vi "CheckCore.vi"(8 "error in (no error)":errorcluster, 9 "# of Refs":i32, 10 "References":refnum<vi>[](array[refnum]), 11 "Function in":refnum<class "Function.lvclass">) -> (0 "error out":errorcluster, 1 "Reject?":bool, 2 "dup References":refnum<vi>[](array[refnum]), 3 "Function out":refnum<class "Function.lvclass">)   [LabVIEW 2014, in "lvbuildsecurity.lvlib" / "Function.lvclass"]
uses:
  Function.lvclass
  Blacklist.lvclass/Blacklist.ctl
  ReadVIRefnum.vi
  ReadCLI.vi
  ReadItems.vi
  <vilib>/Wiresmith Technology/LabVIEW CLI/CLI Class/CLI.lvclass
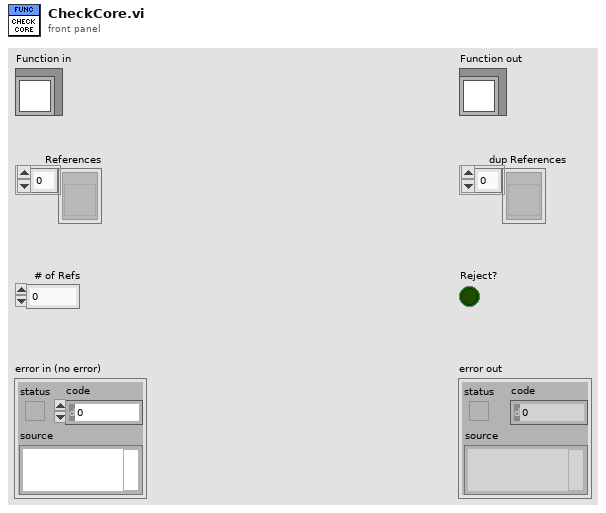
[diagram p1: front panel]
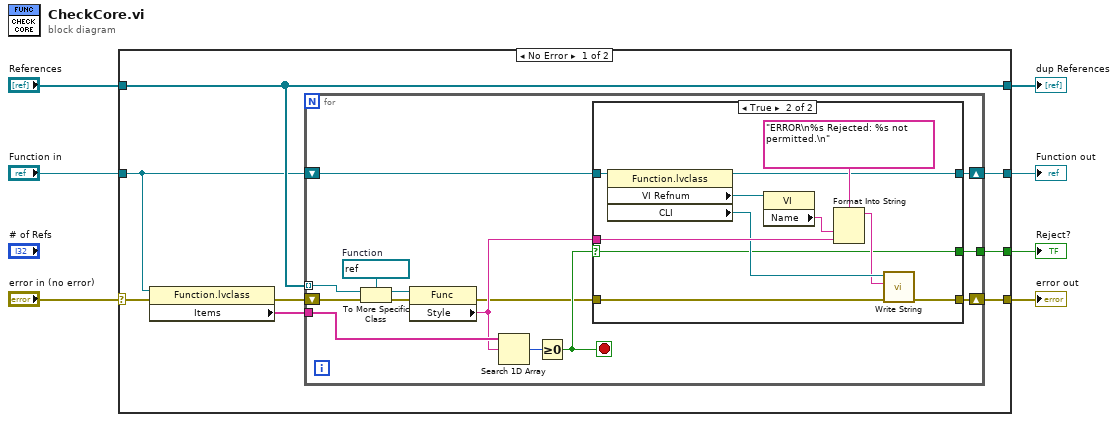
[diagram p0: block diagram]
diagram:
  n1 = case shown="No Error" "error in (no error)" {
    selector: "error in (no error)" -> [w13 w46]
    tunnel: [w15 w46] -> w2
    tunnel: "References" -> [w14 w44]
    tunnel: "Function in" -> [w9 w45]
    tunnel: [w8 w45] -> w6
    tunnel: [w14 w44] -> w5
    tunnel: [w10 _] -> w1
    frame No Error {
      n2 = property class="Function.lvclass"(reference=w9, error in=w13) -> (error out=w12:errorcluster, "Items"=w11:string[])  [unwired: 1 out]
      n3 = for {
        tunnel: w14 -> [w28] mode=indexing
        shift-right: [w17] -> w15
        shift-left: w12 -> [w29]
        tunnel: w11 -> [w24]
        tunnel: [w16] -> w10
        shift-right: [w20] -> w8
        shift-left: w9 -> [w21]
        stop <- w22 stop-if-true
        w27 = refnum<vi> refnum  # Function
        n4 = To More Specific Class(target class=w27, reference=w28, error in=w29) -> (specific class reference=w25:refnum<vi>, error out=w26:errorcluster)
        n5 = property class="Func"(reference=w25, error in=w26) -> (error out=w18:errorcluster, "Style"=w19:string)  [unwired: 1 out]
        n6 = Search 1D Array(1D array=w24, element=w19) -> (index of element=w23:i32)  [unwired: 1 in]
        n7 = Greater Or Equal To 0?(x=w23) -> (x >= 0?=w22:bool)
        n8 = case shown="True" w22 {
          selector: w22 -> [w30 w33]
          tunnel: w21 -> [w32 w43]
          tunnel: [w32 w36] -> w20
          tunnel: w19 -> [_ w39]
          tunnel: w18 -> [w31 w35]
          tunnel: [w31 w34] -> w17
          tunnel: [w30 w33] -> w16
          frame False {
          }
          frame True {
            n9 = property class="Function.lvclass"(reference=w43) -> (reference out=w36:refnum<class "Function.lvclass">, "VI Refnum"=w41:refnum<vi>, "CLI"=w38:refnum<class "CLI.lvclass">)  [unwired: 1 in, 1 out]
            n10 = property class="VI"(reference=w41) -> ("Name"=w40:string)  [unwired: 1 in, 2 out]
            n11 = Format Into String(format string="ERROR\n%s Rejected: %s not permitted.\n", w40, w39) -> (resulting string=w37:string)  [unwired: 2 in, 1 out]
            n12 = call <vilib>:"Write String.vi"("error in (no error)"=w35, "Text to Write"=w37, "CLI in"=w38) -> ("error out"=w34:errorcluster)  [unwired: 7 in, 1 out]
          }
        }
      }
    }
    frame Error {
    }
  }
  "error out" <- w2
  "Function out" <- w6
  "dup References" <- w5
  "Reject?" <- w1
